vi "multichannel.lockin.SMO.vi"() -> ()   [LabVIEW 2016]
uses:
  <vilib>/JKI/JKI SMO/SMO/SMO.lvclass
  <vilib>/JKI/JKI SMO/SMO/Typedefs/SMOState --Enum.ctl
  SMOs/DAQ/DAQ.lvclass
  C:/Program Files (x86)/National Instruments/LabVIEW 2016/vi.lib/JKI/JKI SMO/SMO/SMO.lvclass
  SMOs/DAQmx.AO/DAQmx.AO.lvclass
  SMOs/DAQmx.AI/DAQmx.AI.lvclass
  C:/user/patrick/hg/lockin.SMO/lvsrc/SMOs/DAQmx/DAQmx.lvclass
  C:/user/patrick/hg/lockin.SMO/lvsrc/SMOs/DAQ/DAQ.lvclass
  SMOs/DAQmx/DAQmx.lvclass
  SMOs/lockin/lockin.lvclass
  SMOs/DAQ/Typedefs/SamplingMode.ctl
  SMOs/DAQ/Typedefs/SamplingInfo.ctl
  SMOs/DAQ/Typedefs/PrivateEvents--DAQ.AI.Channels.ctl
  SMOs/DAQ/Typedefs/DAQType.ctl
  SMOs/DAQ/Typedefs/DAQ.Config.ctl
  SMOs/DAQmx.AI/Typedefs/DAQmx.AI.Config.ctl
  SMOs/DAQmx.AO/Typedefs/DAQmx.AO.Config.ctl
panel:
  in  "DAQ.Config (AO)":T1={"Channels"="", "DAQType"=enum."AO", "minimum value"=-5.0, "maximum value"=5.0, "sampling info"={"Fs"=1000.0, "#s"=1000.0}, "SamplingMode"=enum."Continuous", "gain"=[1.0], "offset"=[0.0]} {"offset" format="%0.2f"; "gain" format="%0.2f"; "maximum value" format="%0.2f"; "minimum value" format="%0.2f"}
  in  "DAQmx Physical Channels (AO)":tag="PXI1Slot2/ao0:1, PXI1Slot3/ao0:1, PXI1Slot4/ao0:1, PXI1Slot5/ao0:1"
  in  "DAQmx.AO.config":T6={"output terminal configuration"=-1} {"output terminal configuration" items=["Default"=-1, "RSE"=10083, "Differential"=10106, "Pseudodifferential"=12529]}
  in  "DAQmx.AI.config":T7={"AI.Coupling"=10045, "input terminal configuration "=-1} {"input terminal configuration" items=["default"=-1, "RSE"=10083, "NRSE"=10078, "Differential"=10106, "Pseudodifferential"=12529]; "AI.Coupling" items=["AC"=10045, "DC"=10050, "GND"=10066]}
  in  "DAQmx Physical Channels (AI)":tag="PXI1Slot2/ai0:1, PXI1Slot3/ai0:1, PXI1Slot4/ai0:1, PXI1Slot5/ai0:1"
  in  "DAQ.Config (AI)":T1={"Channels"="", "DAQType"=enum."AI", "minimum value"=-5.0, "maximum value"=5.0, "sampling info"={"Fs"=1000.0, "#s"=1000.0}, "SamplingMode"=enum."Continuous", "gain"=[1.0], "offset"=[0.0]} {"offset" format="%0.2f"; "gain" format="%0.2f"; "maximum value" format="%0.2f"; "minimum value" format="%0.2f"}
  in  "Simulate?":bool
  out "Write":waveform(dbl)[](graph)
  out "Read":T8(graph)
  out "SMO State":T9
  out "error out":errorcluster
  in  "Stop":bool
  # "Multichannel Lockin SMO Test Launcher"
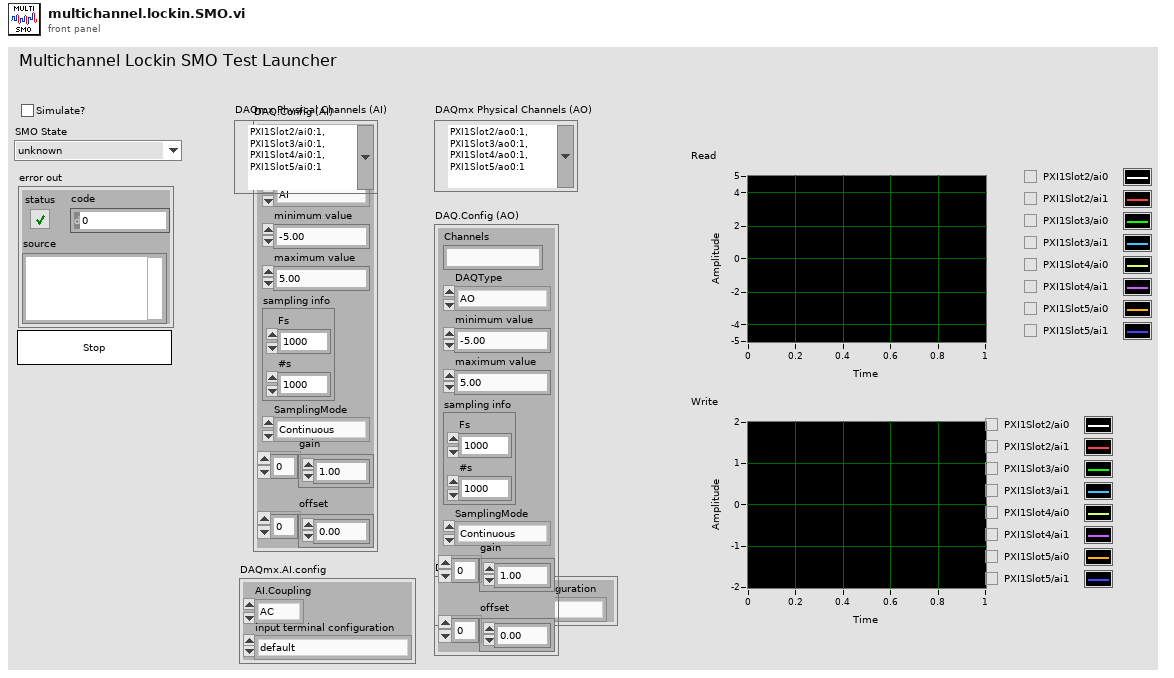
[diagram p1: front panel]
types:
  T1 = typedef "DAQ.lvclass/DAQ.Config.ctl" = cluster{"Channels":T2, "DAQType":T3, "minimum value":dbl, "maximum value":dbl, "sampling info":T4, "SamplingMode":T5, "gain":dbl[], "offset":dbl[]}
  T2 = typedef "DAQ.lvclass/PrivateEvents--DAQ.AI.Channels.ctl" = string
  T3 = typedef "DAQ.lvclass/DAQType.ctl" = enum16{"AI", "AO"}
  T4 = typedef "DAQ.lvclass/SamplingInfo.ctl" = cluster{"Fs":dbl, "#s":dbl}
  T5 = typedef "DAQ.lvclass/SamplingMode.ctl" = enum16{"Continuous", "Finite"}
  T6 = typedef "DAQmx.AO.lvclass/DAQmx.AO.Config.ctl" = cluster{"output terminal configuration":i32}
  T7 = typedef "DAQmx.AI.lvclass/DAQmx.AI.Config.ctl" = cluster{"AI.Coupling":i32, "input terminal configuration ":i32}
  T8 = typedef "DAQ.lvclass/PublicEvents--DAQ.Read.ctl" = waveform(dbl)[]
  T9 = typedef "SMO.lvclass/SMOState --Enum.ctl" = enum16{"unknown", "Created", "Started", "Stopped"}
  T10 = typedef "SMO.lvclass/Public Events.ctl" = cluster{"Error":refnum<user-event>, "State":refnum<user-event>, "Reserve State":refnum<user-event>}
  T11 = typedef "DAQ.lvclass/PublicEvents--Cluster.ctl" = cluster{"Read":refnum<user-event>, "Write":refnum<user-event>}
  T12 = typedef "DAQ.lvclass/PublicEvents--DAQ.Write.ctl" = waveform(dbl)[]
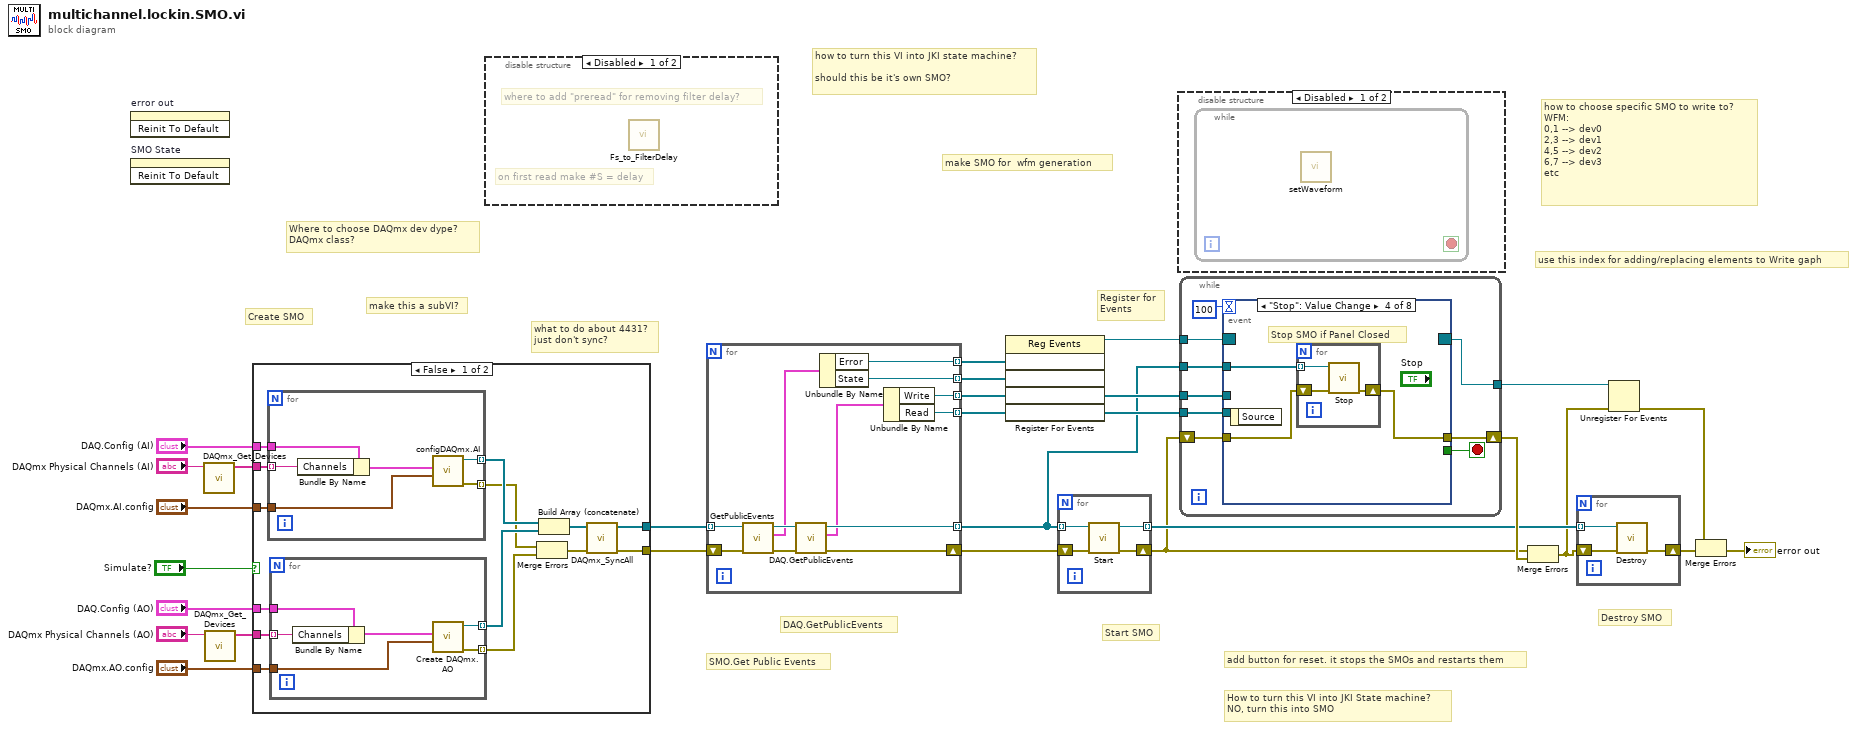
[diagram p0: block diagram]
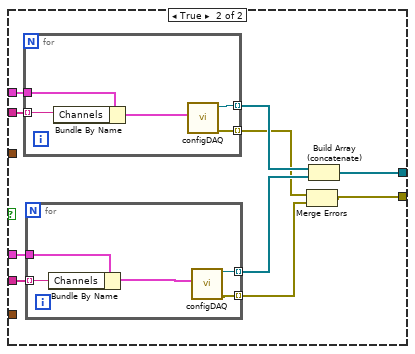
[diagram p4: hidden frame]
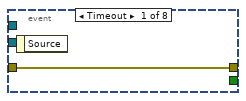
[diagram p5: hidden frame]
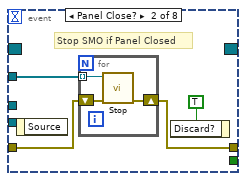
[diagram p6: hidden frame]
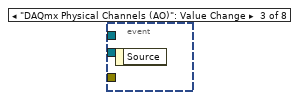
[diagram p7: hidden frame]
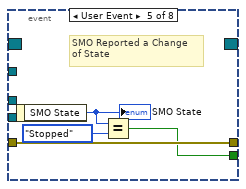
[diagram p8: hidden frame]
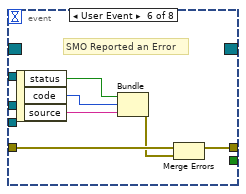
[diagram p9: hidden frame]
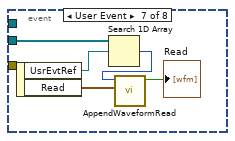
[diagram p10: hidden frame]
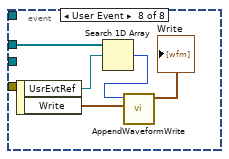
[diagram p11: hidden frame]
diagram:
  # "How to turn this VI into JKI State machine?\nNO, turn this into SMO"
  # "add button for reset. it stops the SMOs and restarts them"
  # "how to turn this VI into JKI state machine?\n\nshould this be it's own SMO?"
  # "Where to choose DAQmx dev dype?\nDAQmx class?"
  # "what to do about 4431?\njust don't sync?"
  # "make this a subVI?"
  # "how to choose specific SMO to write to?\nWFM:\n0,1 --> dev0\n2,3 --> dev1\n4,5 --> dev2\n6,7 --> dev3\netc"
  # "use this index for adding/replacing elements to Write gaph"
  # "make SMO for  wfm generation"
  # "DAQ.GetPublicEvents"
  # "SMO.Get Public Events"
  # "Start SMO"
  # "Destroy SMO"
  # "Create SMO"
  # "Register for Events"
  n1 = invoke on="error out" class="Clust (strict)" method="Reinit To Default"() -> ()  [unwired: 3 in, 3 out]
  n2 = invoke on="SMO State" class="Enum (strict)" method="Reinit To Default"() -> ()  [unwired: 3 in, 3 out]
  n3 = call "DAQmx_Get_Devices.vi"("DAQmx Physical Channel"="DAQmx Physical Channels (AI)") -> ("Channels Array"=w15:string[])  [unwired: 10 in]
  n4 = call "DAQmx_Get_Devices.vi"("DAQmx Physical Channel"="DAQmx Physical Channels (AO)") -> ("Channels Array"=w12:string[])  [unwired: 10 in]
  n5 = case shown="False" "Simulate?" {
    tunnel: "DAQ.Config (AO)" -> [w40 w62]
    tunnel: "DAQmx.AO.config" -> [w39 _]
    tunnel: w15 -> [w38 w61]
    tunnel: "DAQ.Config (AI)" -> [w37 w60]
    tunnel: "DAQmx.AI.config" -> [w36 _]
    tunnel: w12 -> [w35 w59]
    tunnel: [w30 w53] -> w11
    tunnel: [w29 w54] -> w10
    frame False {
      n6 = for {
        tunnel: w38 -> [w52] mode=indexing
        tunnel: w37 -> [w51]
        tunnel: w36 -> [w49]
        tunnel: [w48] -> w32 mode=indexing
        tunnel: [w47] -> w34 mode=indexing
        n7 = Bundle By Name(cluster=w51, "Channels"=w52) -> (w50:T1)
        n8 = call "configDAQmx.AI.vi"("DAQmx.AI.config"=w49, "DAQ.config"=w50) -> ("error out"=w48:errorcluster, "DAQmx.AI out"=w47:refnum<class "DAQmx.AI.lvclass">)  [unwired: 8 in]
      }
      n9 = for {
        tunnel: w40 -> [w46]
        tunnel: w39 -> [w43]
        tunnel: w35 -> [w44] mode=indexing
        tunnel: [w42] -> w33 mode=indexing
        tunnel: [w41] -> w31 mode=indexing
        n10 = Bundle By Name(cluster=w46, "Channels"=w44) -> (w45:T1)
        n11 = call "Create DAQmx.AO.vi"("DAQmx.AO.config"=w43, "DAQ.Config"=w45) -> ("error out"=w41:errorcluster, "DAQmx.AO out"=w42:refnum<class "DAQmx.AO.lvclass">)  [unwired: 8 in]
      }
      n12 = Merge Errors(w32, w31) -> (w27:errorcluster)
      n13 = Build Array (concatenate)(w34, w33) -> (w28:refnum<class "DAQmx.lvclass">[])
      n14 = call "DAQmx_SyncAll.vi"("error in (no error)"=w27, "Array in"=w28) -> ("error out"=w30:errorcluster, "Array out"=w29:refnum<class "DAQmx.lvclass">[])  [unwired: 8 in]
    }
    frame True {
      n15 = for {
        tunnel: w61 -> [w72] mode=indexing
        tunnel: w60 -> [w71]
        tunnel: [w68] -> w56 mode=indexing
        tunnel: [w69] -> w58 mode=indexing
        n16 = Bundle By Name(cluster=w71, "Channels"=w72) -> (w70:T1)
        n17 = call "configDAQ.vi"("DAQ.Config"=w70) -> ("error out"=w68:errorcluster, "DAQ out"=w69:refnum<class "DAQ.lvclass">)  [unwired: 9 in]
      }
      n18 = for {
        tunnel: w62 -> [w67]
        tunnel: w59 -> [w66] mode=indexing
        tunnel: [w65] -> w57 mode=indexing
        tunnel: [w64] -> w55 mode=indexing
        n19 = Bundle By Name(cluster=w67, "Channels"=w66) -> (w63:T1)
        n20 = call "configDAQ.vi"("DAQ.Config"=w63) -> ("error out"=w64:errorcluster, "DAQ out"=w65:refnum<class "DAQ.lvclass">)  [unwired: 9 in]
      }
      n21 = Merge Errors(w56, w55) -> (w53:errorcluster)
      n22 = Build Array (concatenate)(w58, w57) -> (w54:refnum<class "DAQ.lvclass">[])
    }
  }
  n23 = disable-structure shown="Disabled" {
    frame Disabled {
      # "on first read make #S = delay"
      # "where to add \"preread\" for removing filter delay?"
      n24 = call "Fs_to_FilterDelay.vi"() -> ()  [unwired: 11 in, 1 out]
    }
    frame Enabled {
    }
  }
  n25 = for {
    tunnel: [w83] -> w1 mode=indexing
    tunnel: w10 -> [w82] mode=indexing
    shift-right: [w79] -> w20
    shift-left: w11 -> [w81]
    tunnel: [w78] -> w3 mode=indexing
    tunnel: [w76] -> w2 mode=indexing
    tunnel: [w74] -> w7 mode=indexing
    tunnel: [w73] -> w6 mode=indexing
    n26 = call <vilib>:"GetPublicEvents.vi"("error in (no error)"=w81, "SMO"=w82) -> ("error out"=w84:errorcluster, "Public Events"=w75:T10, "SMO out"=w80:refnum<class "DAQ.lvclass">)  [unwired: 7 in]
    n27 = call "DAQ.GetPublicEvents.vi"("error in (no error)"=w84, "DAQ"=w80) -> ("error out"=w79:errorcluster, "Public Events"=w77:T11, "DAQ out"=w83:refnum<class "DAQ.lvclass">)  [unwired: 7 in]
    n28 = Unbundle By Name(w75) -> ("Error"=w73:refnum<user-event>, "State"=w74:refnum<user-event>)
    n29 = Unbundle By Name(w77) -> ("Write"=w78:refnum<user-event>, "Read"=w76:refnum<user-event>)
  }
  n30 = register-events(w6, w7, w3, w2) -> (reference out=w5:refnum<event-registration>)  [unwired: 2 in, 1 out]
  n31 = for {
    shift-right: [w87] -> w21
    shift-left: w20 -> [w85]
    tunnel: w1 -> [w86] mode=indexing
    tunnel: [w88] -> w22 mode=indexing
    n32 = call <vilib>:"Start.vi"("error in (no error)"=w85, "SMO"=w86) -> ("error out"=w87:errorcluster, "SMO out"=w88:refnum<class "DAQ.lvclass">)  [unwired: 8 in]
  }
  n33 = disable-structure shown="Disabled" {
    frame Disabled {
      n34 = while {
        stop <- _ stop-if-true
        n35 = call "setWaveform.vi"() -> ()  [unwired: 10 in, 2 out]
      }
    }
    frame Enabled {
    }
  }
  n36 = while {
    shift-right: [w96] -> w26
    shift-left: w21 -> [w95]
    tunnel: w5 -> [w94]
    tunnel: [w93] -> w4
    tunnel: w1 -> [w91]
    tunnel: w3 -> [w90]
    tunnel: w2 -> [w89]
    stop <- w97 stop-if-true
    n37 = event shown="[3] \"Stop\": Value Change" {
      selector: w94 -> [_ _ _ _ _ _ _ _]
      dyn-events: [_ _ _ _ _ _ _ _] -> w93
      timeout: 100 -> [_ _ _ _ _ _ _ _]
      tunnel: [_ _ _ _ w112 _ _ _] -> w97
      tunnel: [w98 w102 _ w108 w115 w119 _ _] -> w96
      tunnel: w95 -> [w98 w99 _ w107 w115 w117 _ _]
      tunnel: w91 -> [_ w100 _ w106 _ _ _ _]
      tunnel: w90 -> [_ _ _ _ _ _ _ w131]
      tunnel: w89 -> [_ _ _ _ _ _ w126 _]
      event Timeout {
        n38 = event-data() -> ()  [unwired: 1 in, 1 out]
      }
      event Panel Close? {
        # "Stop SMO if Panel Closed"
        n39 = event-data() -> ()  [unwired: 1 in, 1 out]
        n40 = for {
          shift-right: [w105] -> w102
          shift-left: w99 -> [w104]
          tunnel: w100 -> [w103] mode=indexing
          n41 = call <vilib>:"Stop.vi"("error in (no error)"=w104, "SMO"=w103) -> ("error out"=w105:errorcluster)  [unwired: 8 in, 1 out]
        }
        n42 = event-data("Discard?"=TRUE ("OK")) -> ()  [unwired: 1 in, 1 out]
      }
      event "DAQmx Physical Channels (AO)": Value Change {
        n43 = event-data() -> ()  [unwired: 1 in, 1 out]
      }
      event "Stop": Value Change {
        # "Stop SMO if Panel Closed"
        n44 = event-data() -> ()  [unwired: 1 in, 1 out]
        n45 = for {
          shift-right: [w111] -> w108
          shift-left: w107 -> [w110]
          tunnel: w106 -> [w109] mode=indexing
          n46 = call <vilib>:"Stop.vi"("error in (no error)"=w110, "SMO"=w109) -> ("error out"=w111:errorcluster)  [unwired: 8 in, 1 out]
        }
      }
      event User Event {
        # "SMO Reported a Change\nof State"
        n47 = event-data() -> ("SMO State"=w114:T9)  [unwired: 1 in]
        "SMO State" <- w114
        n48 = Equal?(x=w114, y=SMOState_--Enum."Stopped") -> (x = y?=w112:bool)
      }
      event User Event {
        # "SMO Reported an Error"
        n49 = event-data() -> ("status"=w118:bool, "code"=w121:i32, "source"=w120:string)  [unwired: 1 in]
        n50 = Bundle("status"=w118, "code"=w121, "source"=w120) -> (w116:errorcluster)  [unwired: 1 in]
        n51 = Merge Errors(w117, w116) -> (w119:errorcluster)
      }
      event User Event {
        n52 = event-data() -> ("UsrEvtRef"=w125:refnum<user-event>, "Read"=w124:T8)  [unwired: 1 in]
        n53 = Search 1D Array(1D array=w126, element=w125) -> (index of element=w122:i32)  [unwired: 1 in]
        n54 = call "AppendWaveformRead.vi"("WFM in"=w124, "index of element"=w122) -> ("x = y?"=→"Read":bool)  [unwired: 8 in, 1 out]
      }
      event User Event {
        n55 = event-data() -> ("UsrEvtRef"=w130:refnum<user-event>, "Write"=w129:T12)  [unwired: 1 in]
        n56 = Search 1D Array(1D array=w131, element=w130) -> (index of element=w127:i32)  [unwired: 1 in]
        n57 = call "AppendWaveformWrite.vi"("WFM in in"=w129, "index of element"=w127) -> ("WFM out"=→"Write":T12)  [unwired: 9 in]
      }
    }
  }
  n58 = Merge Errors(w21, w26) -> (w8:errorcluster)
  n59 = for {
    tunnel: w22 -> [w132] mode=indexing
    shift-right: [w134] -> w23
    shift-left: w8 -> [w133]
    n60 = call <vilib>:"Destroy.vi"("error in (no error)"=w133, "SMO"=w132) -> ("error out"=w134:errorcluster)  [unwired: 9 in]
  }
  n61 = Unregister For Events(event registration refnum=w4, error in=w8) -> (error out=w25:errorcluster)
  n62 = Merge Errors(w25, w23) -> (→"error out":errorcluster)
